vi "GetCiscoStats(SubVI).vi"(8 "error in (no error)":errorcluster) -> (0 "error IO":errorcluster, 2 "Valid Data ?":bool, 3 "Cisco Stats":T1[](array[typedef]))   [LabVIEW 2017, in "MainFrameLib.lvlib"]
uses:
  MainFrameLib.lvlib
  TypeDefs/CiscoStats.ctl
  <vilib>/httpClient/LabVIEWHTTPClient.lvlib
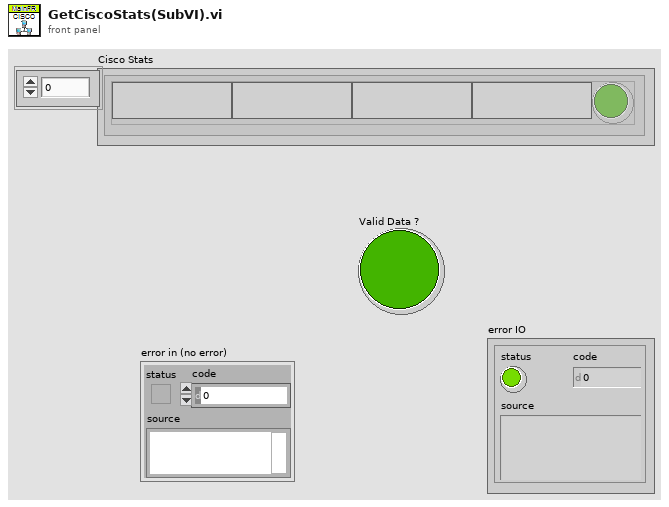
[diagram p1: front panel]
types:
  T1 = typedef "MainFrameLib.lvlib/CiscoStats.ctl" = cluster{"Agent Name":string, "Number":string, "State":string, "Time in state":string, "Ready ?":bool}
  T2 = typedef "LabVIEWHTTPClient.lvlib/ClientHandle.ctl" = refnum<k1>
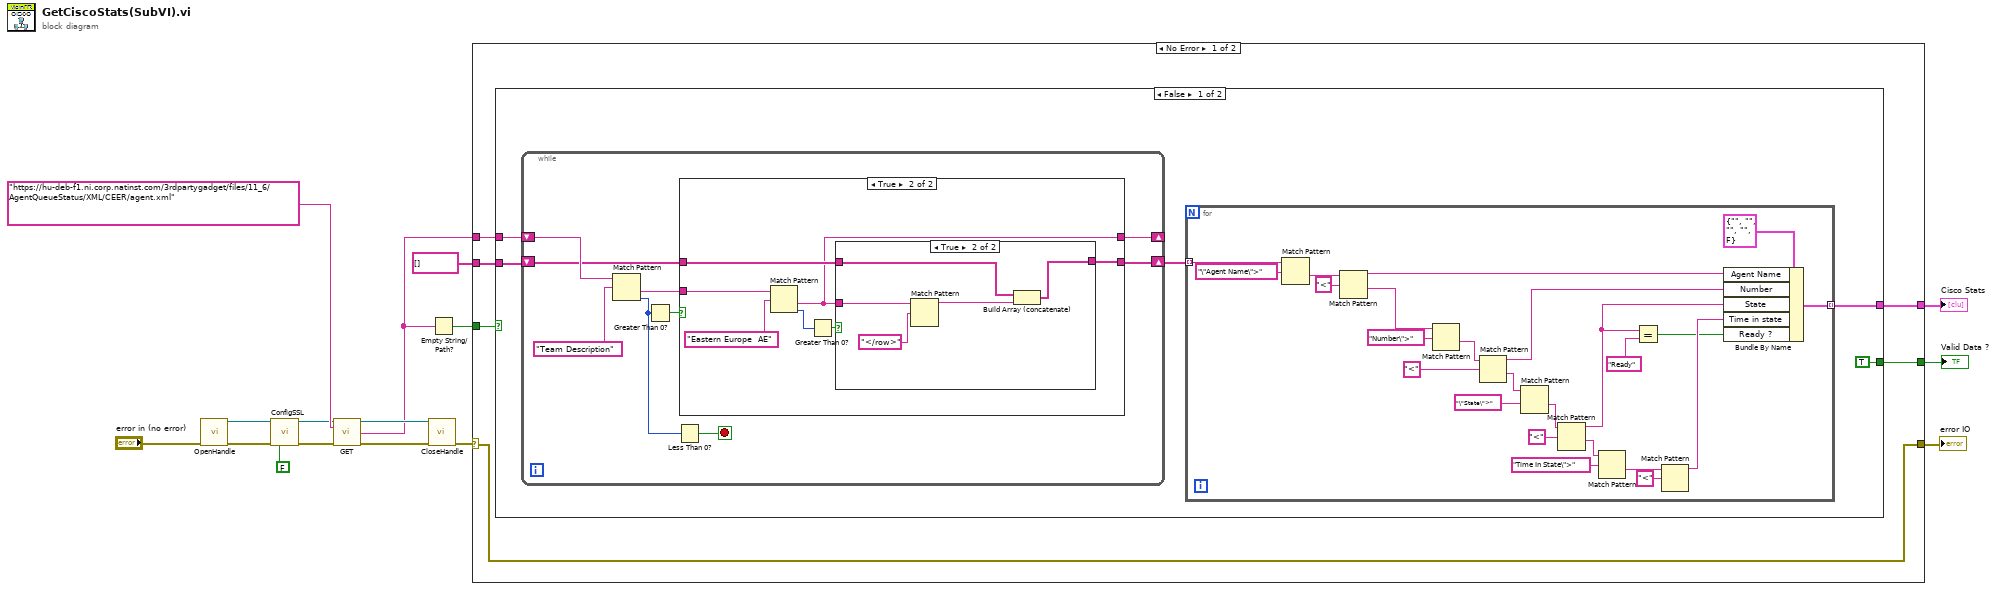
[diagram p0: block diagram]
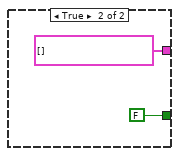
[diagram p4: hidden frame]
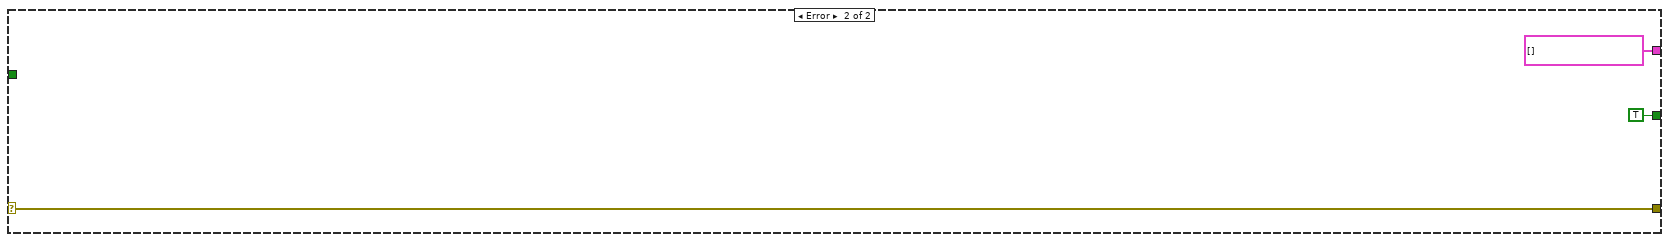
[diagram p5: hidden frame]
diagram:
  n1 = call <vilib>:"OpenHandle.vi"("error in (no error)"="error in (no error)") -> ("client handle out"=w2:T2, "error out"=w5:errorcluster)  [unwired: 13 in]
  n2 = call <vilib>:"ConfigSSL.vi"("client handle"=w2, "error in (no error)"=w5, "verify server (true)"=FALSE) -> ("client handle out"=w1:T2, "error out"=w4:errorcluster)  [unwired: 11 in]
  n3 = call <vilib>:"GET.vi"("client handle"=w1, "url"="https://hu-deb-f1.ni.corp.natinst.com/3rdpartygadget/files/11_6/AgentQueueStatus/XML/CEER/agent.xml" ("URL"), "error in (no error)"=w4) -> ("client handle out"=w14:T2, "body"=w8:string, "error out"=w15:errorcluster)  [unwired: 9 in, 1 out]
  n4 = call <vilib>:"CloseHandle.vi"("client handle"=w14, "error in (no error)"=w15) -> ("error out"=w12:errorcluster)  [unwired: 13 in]
  n5 = Empty String/Path?(string/path=w8) -> (empty?=w13:bool)
  n6 = case shown="No Error" w12 {
    selector: w12 -> [w17 w79]
    tunnel: [w22 T1[] []] -> w6
    tunnel: w13 -> [w21 _]
    tunnel: [w20 TRUE] -> w11
    tunnel: [w17 w79] -> w9
    tunnel: w8 -> [w19 _]
    tunnel: string[] [] -> [w18 _]
    frame No Error {
      n7 = case shown="False" w21 {
        tunnel: [w27 T1[] []] -> w22
        tunnel: [TRUE FALSE] -> w20
        tunnel: w19 -> [w25 _]
        tunnel: w18 -> [w24 _]
        frame False {
          n8 = while {
            shift-right: [w28] -> _
            shift-left: w25 -> [w35]
            shift-right: [w30] -> w26
            shift-left: w24 -> [w29]
            stop <- w34 stop-if-true
            n9 = Match Pattern(string=w35, regular expression="Team Description") -> (after substring=w31:string, offset past match=w33:i32)  [unwired: 1 in, 2 out]
            n10 = Greater Than 0?(x=w33) -> (x > 0?=w32:bool)
            n11 = Less Than 0?(x=w33) -> (x < 0?=w34:bool)
            n12 = case shown="True" w32 {
              tunnel: w31 -> [w37 w45]
              tunnel: [w38 w41] -> w30
              tunnel: w29 -> [w38 w40]
              tunnel: [w37 w39] -> w28
              frame False {
              }
              frame True {
                n13 = Match Pattern(string=w45, regular expression="Eastern Europe  AE") -> (after substring=w39:string, offset past match=w43:i32)  [unwired: 1 in, 2 out]
                n14 = Greater Than 0?(x=w43) -> (x > 0?=w42:bool)
                n15 = case shown="True" w42 {
                  tunnel: w39 -> [_ w51]
                  tunnel: [w46 w48] -> w41
                  tunnel: w40 -> [w46 w47]
                  frame False {
                  }
                  frame True {
                    n16 = Match Pattern(string=w51, regular expression="</row>") -> (before substring=w49:string)  [unwired: 1 in, 3 out]
                    n17 = Build Array (concatenate)(w47, w49) -> (w48:string[])
                  }
                }
              }
            }
          }
          n18 = for {
            tunnel: w26 -> [w61] mode=indexing
            tunnel: [w62] -> w27 mode=indexing
            n19 = Match Pattern(string=w61, regular expression="\"Agent Name\">") -> (after substring=w74:string)  [unwired: 1 in, 3 out]
            n20 = Match Pattern(string=w74, regular expression="<") -> (before substring=w72:string, after substring=w59:string)  [unwired: 1 in, 2 out]
            n21 = Match Pattern(string=w59, regular expression="Number\">") -> (after substring=w60:string)  [unwired: 1 in, 3 out]
            n22 = Match Pattern(string=w60, regular expression="<") -> (before substring=w69:string, after substring=w58:string)  [unwired: 1 in, 2 out]
            n23 = Match Pattern(string=w58, regular expression="\"State\">") -> (after substring=w55:string)  [unwired: 1 in, 3 out]
            n24 = Match Pattern(string=w55, regular expression="<") -> (before substring=w52:string, after substring=w57:string)  [unwired: 1 in, 2 out]
            n25 = Match Pattern(string=w57, regular expression="Time In State\">") -> (after substring=w65:string)  [unwired: 1 in, 3 out]
            n26 = Equal?(x=w52, y="Ready") -> (x = y?=w53:bool)
            n27 = Match Pattern(string=w65, regular expression="<") -> (before substring=w63:string)  [unwired: 1 in, 3 out]
            n28 = Bundle By Name(cluster=T1 {"Agent Name"="", "Number"="", "State"="", "Time in state"="", "Ready ?"=FALSE} ("Cluster"), "Agent Name"=w72, "Number"=w69, "State"=w52, "Time in state"=w63, "Ready ?"=w53) -> (w62:T1)
          }
        }
        frame True {
        }
      }
    }
    frame Error {
    }
  }
  "Valid Data ?" <- w11
  "error IO" <- w9
  "Cisco Stats" <- w6
